vi "Close stdin.vi"(11 "subprocess in":refnum<class "Buffered Subprocess.lvclass">) -> (3 "subprocess out":refnum<class "Buffered Subprocess.lvclass">)   [LabVIEW 2020, in "NI_Subprocess.lvlib" / "Buffered Subprocess.lvclass"]
uses:
  <vilib>/Subprocess/Buffered Subprocess/Buffered Subprocess.lvclass
  <vilib>/Subprocess/Buffered Subprocess/Buffered Subprocess.lvclass/Buffered Subprocess.ctl
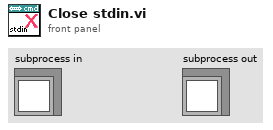
[diagram p1: front panel]
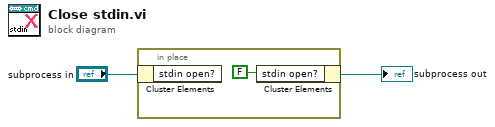
[diagram p0: block diagram]
diagram:
  n1 = in-place {
    n2 = in-place-cluster #1("subprocess in") -> ()  [unwired: 1 out]
    n3 = in-place-cluster #1("stdin open?"=FALSE) -> (→"subprocess out":refnum<class "Buffered Subprocess.lvclass">)
  }
